vi "EventClient_Flush.vi"(8 "error in (no error)":errorcluster, 11 "reference":T1) -> (0 "error out":errorcluster, 3 "reference out":T1)   [LabVIEW 2018]
uses:
  EventClient_ObjectReference.ctl
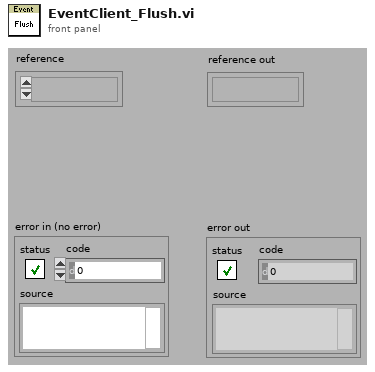
[diagram p1: front panel]
types:
  T1 = typedef "EventClient_ObjectReference.ctl" = refnum<k1>
  T2 = cluster{"Client":refnum<queue>, "Sub Events":string[], "PrvData":variant, "MyName":string}
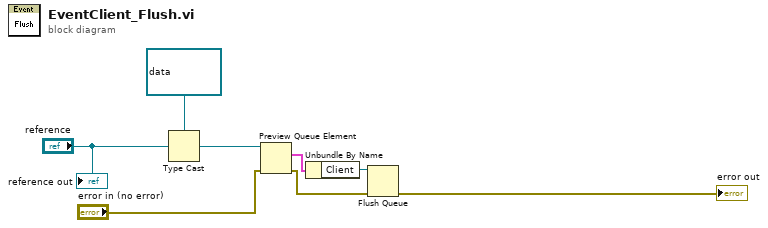
[diagram p0: block diagram]
diagram:
  n1 = Type Cast(type=refnum<queue> refnum ("queue out"), x="reference") -> (*(type *) &x=w7:refnum<queue>)
  n2 = Preview Queue Element(queue=w7, error in (no error)="error in (no error)") -> (element=w6:T2, error out=w2:errorcluster)  [unwired: 3 out]
  n3 = Unbundle By Name(w6) -> ("Client"=w4:refnum<queue>)
  n4 = Flush Queue(queue=w4, error in (no error)=w2) -> (error out=→"error out":errorcluster)  [unwired: 2 out]
  "reference out" <- "reference"
